vi "Close.vi"(8 "error in":errorcluster, 11 "Actual Value in":refnum<class "Actual Value.lvclass">) -> (0 "error out":errorcluster, 3 "Actual Value out":refnum<class "Actual Value.lvclass">)   [LabVIEW 2023, in "Actual Value.lvclass"]
uses:
  Actual Value.lvclass
  Actual Value.lvclass/Actual Value.ctl
  <vilib>/ADAS Replay HIL/AdasHilServices/AdasHilChannelServices.lvlib
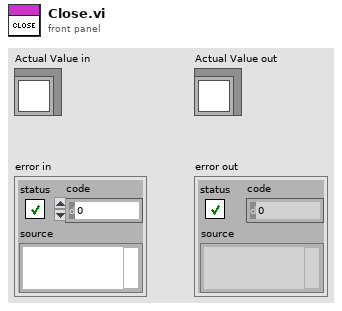
[diagram p1: front panel]
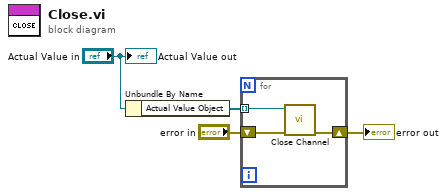
[diagram p0: block diagram]
diagram:
  n1 = Unbundle By Name("Actual Value in") -> ("Actual Value Object"=w4:refnum<k21>[])
  n2 = for {
    tunnel: w4 -> [w5] mode=indexing
    shift-right: [w7] -> w2
    shift-left: "error in" -> [w6]
    n3 = call <vilib>:"Close Channel.vi"("error in"=w6, "ADAS HIL Channel"=w5) -> ("error out"=w7:errorcluster)  [unwired: 9 in]
  }
  "error out" <- w2
  "Actual Value out" <- "Actual Value in"
